vi "INI Read write DblArry.vi"(5 "key":string, 7 "section":string, 8 "error in":errorcluster, 9 "default":dbl[](array[numeric]) format="%.2f", 10 "dbl array in":dbl[](array[numeric]) format="%.2f", 11 "Read|Write":T1) -> (0 "error out":errorcluster, 2 "dbl array out":dbl[](array[numeric]) format="%.2f")   [LabVIEW 2013]
doc: "This .vi reads/writes a double to the config file. During Write, \"dbl in\" is passed to \"dbl out\""
uses:
  Read write mode.ctl
  <vilib>/Utility/config.llb/Read Key (String).vi
  <vilib>/Utility/config.llb/Write Key (String).vi
  <vilib>/Utility/config.llb/NI_LVConfig.lvlib
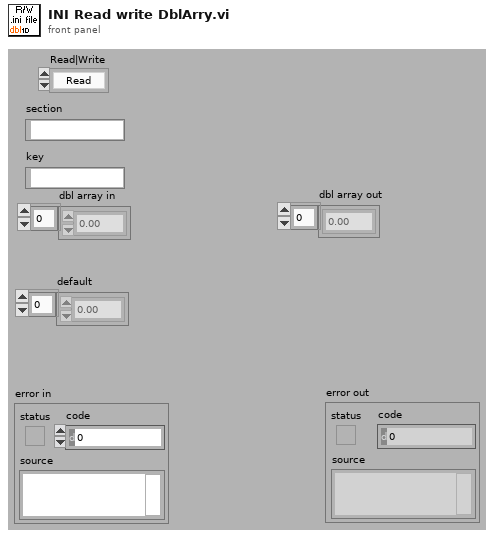
[diagram p1: front panel]
types:
  T1 = typedef "Read write mode.ctl" = enum16{"Read", "Write"}
  T2 = typedef "Semaphore RefNum" = refnum<k1>
  T3 = typedef "NI_LVConfig.lvlib/Config Data RefNum.ctl" = refnum<k1>
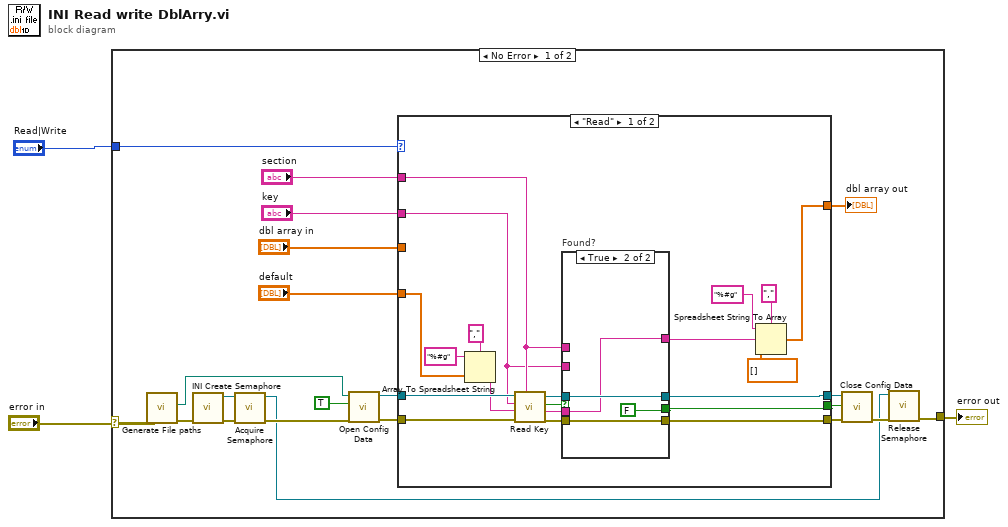
[diagram p0: block diagram]
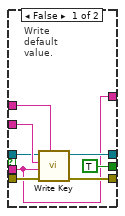
[diagram p2: hidden frame]
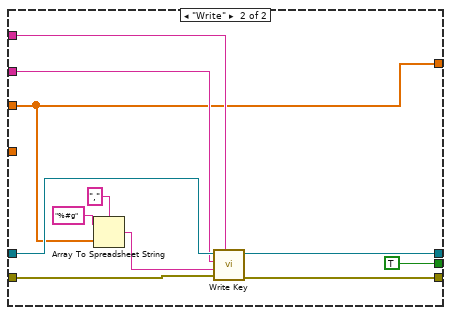
[diagram p3: hidden frame]
diagram:
  n1 = case shown="No Error" "error in" {
    selector: "error in" -> [_ w67]
    tunnel: "Read|Write" -> [w23 _]
    tunnel: [w6 w67] -> w1
    frame No Error {
      n2 = call "Generate File paths.vi"() -> ("error out"=w5:errorcluster, ".ini path"=w4:path)  [unwired: 1 in, 9 out]
      n3 = call "INI Create Semaphore.vi"("error in"=w5) -> ("error out"=w11:errorcluster, "semaphore"=w10:T2)  [unwired: 1 in, 4 out]
      n4 = call <vilib>:"Acquire Semaphore.vi"("error in (no error)"=w11, "semaphore"=w10) -> ("error out"=w9:errorcluster, "semaphore out"=w7:T2)  [unwired: 1 in, 3 out]
      n5 = call <vilib>:"Open Config Data.vi"("error in (no error)"=w9, "create file if necessary (T)"=TRUE ("create file if necessary? (T)"), "configuration file path"=w4) -> ("error out"=w18:errorcluster, "refnum"=w21:T3)  [unwired: 6 in, 1 out]
      n6 = case shown="\"Read\"" w23 {
        tunnel: [w40 w65] -> w20
        tunnel: w21 -> [w43 w66]
        tunnel: [w36 w64] -> w19
        tunnel: w18 -> [w42 w56]
        tunnel: "section" -> [w39 w63]
        tunnel: "key" -> [w38 w62]
        tunnel: [w29 w59] -> w15
        tunnel: "dbl array in" -> [_ w59]
        tunnel: [w34 TRUE ("write configuration file? (T)")] -> w13
        tunnel: "default" -> [w26 _]
        frame "Read" {
          n7 = Array To Spreadsheet String(delimiter (Tab)=",", array=w26, 3:"%#g" ("format string")) -> (spreadsheet string=w25:string)
          n8 = call-poly <vilib>:"Read Key.vi"("section"=w39, "error in (no error)"=w42, "default value"=w25, "key"=w38, "refnum"=w43) -> ("error out"=w41:errorcluster, "value"=w33:string, "found?"=w37:bool, "refnum out"=w35:T3)  [unwired: 1 in, 2 out]
          n9 = case "Found?" shown="True" w37 {
            tunnel: w41 -> [w51 w55]
            tunnel: [w50 w55] -> w40
            tunnel: w35 -> [w46 w54]
            tunnel: [w49 w54] -> w36
            tunnel: w39 -> [w48 _]
            tunnel: w38 -> [w47 _]
            tunnel: [TRUE ("write configuration file? (T)") FALSE ("write configuration file? (T)")] -> w34
            tunnel: w33 -> [w44 w52]
            tunnel: [w44 w52] -> w24
            frame False {
              # "Write\ndefault\nvalue."
              n10 = call-poly <vilib>:"Write Key.vi"("section"=w48, "error in (no error)"=w51, "value"=w44, "key"=w47, "refnum"=w46) -> ("error out"=w50:errorcluster, "refnum out"=w49:T3)  [unwired: 1 in, 4 out]
            }
            frame True {
            }
          }
          n11 = Spreadsheet String To Array(delimiter (Tab)=",", format string="%#g", spreadsheet string=w24, array type (2D Dbl)=dbl[] []) -> (array=w29:dbl[])
        }
        frame "Write" {
          n12 = Array To Spreadsheet String(delimiter (Tab)=",", array=w59, 3:"%#g" ("format string")) -> (spreadsheet string=w57:string)
          n13 = call-poly <vilib>:"Write Key.vi"("section"=w63, "error in (no error)"=w56, "value"=w57, "key"=w62, "refnum"=w66) -> ("error out"=w65:errorcluster, "refnum out"=w64:T3)  [unwired: 1 in, 4 out]
        }
      }
      "dbl array out" <- w15
      n14 = call <vilib>:"Close Config Data.vi"("error in (no error)"=w20, "write file if changed (T)"=w13, "refnum"=w19) -> ("error out"=w8:errorcluster)  [unwired: 8 out]
      n15 = call <vilib>:"Release Semaphore.vi"("error in (no error)"=w8, "semaphore"=w7) -> ("error out"=w6:errorcluster)  [unwired: 5 out]
    }
    frame Error {
    }
  }
  "error out" <- w1
